vi "whileState.vi"(8 "error in (no error)":errorcluster, 11 "unknown in":refnum<class "unknown.lvclass">) -> (0 "error out":errorcluster, 1 "Done?":bool, 2 "next state":refnum<class "state.lvclass">, 3 "unknown out":refnum<class "unknown.lvclass">)   [LabVIEW 2020, in "eos.lvlib" / "unknown.lvclass"]
uses:
  unknown.lvclass
  interfaces/state/state.lvclass
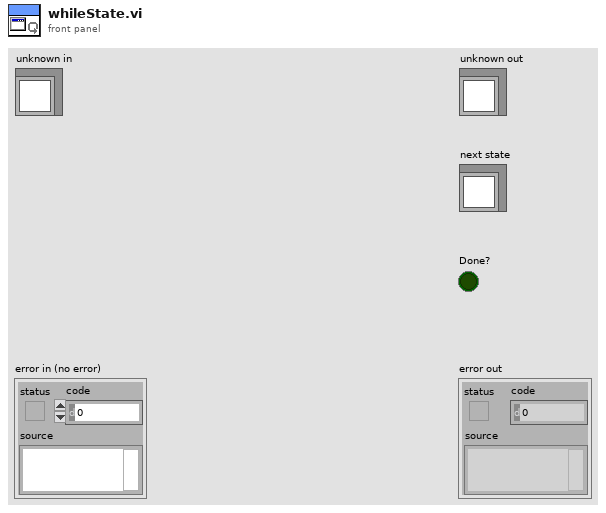
[diagram p1: front panel]
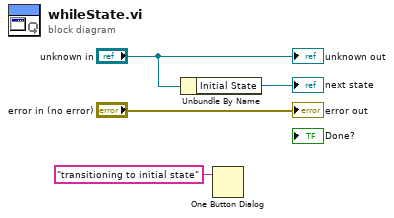
[diagram p0: block diagram]
diagram:
  n1 = Unbundle By Name("unknown in") -> ("Initial State"=→"next state":refnum<class "state.lvclass">)
  n2 = One Button Dialog(message="transitioning to initial state") -> ()  [unwired: 1 in, 1 out]
  "error out" <- "error in (no error)"
  "unknown out" <- "unknown in"
